vi "Read Initial variables.vi"(8 "error in (no error)":errorcluster, 11 "Channel in":refnum<class "Channel.lvclass">) -> (0 "error out":errorcluster, 2 "Initial variables":T1, 3 "Channel out":refnum<class "Channel.lvclass">)   [LabVIEW 2018]
uses:
  Channel.lvclass
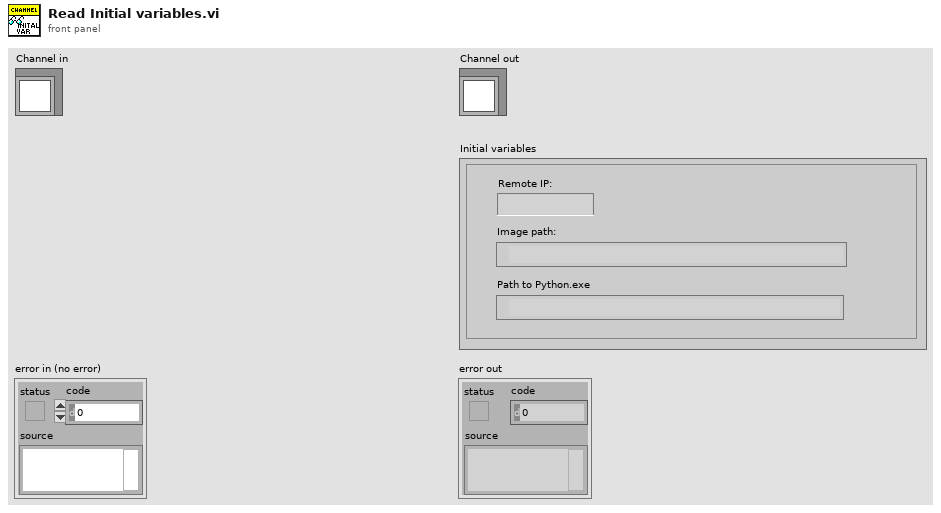
[diagram p1: front panel]
types:
  T1 = cluster{"Image path:":path, "Remote IP:":string, "Path to Python.exe":path}
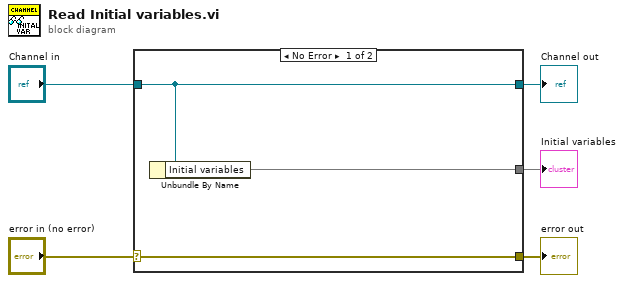
[diagram p0: block diagram]
diagram:
  n1 = case shown="No Error" "error in (no error)" {
    selector: "error in (no error)" -> [w8 w9]
    tunnel: [w8 w9] -> w4
    tunnel: [w7 w10] -> w2
    tunnel: "Channel in" -> [w7 w10]
    tunnel: [w6 _] -> w1
    frame No Error {
      n2 = Unbundle By Name(w7) -> ("Initial variables"=w6)
    }
    frame Error {
    }
  }
  "error out" <- w4
  "Channel out" <- w2
  "Initial variables" <- w1
